vi "ATF-Sample Rate.vi"(10 "Sample Rate":T2, 11 "Device List":T3) -> ()   [LabVIEW 2022 SP3]
panel:
  out "SR":T1
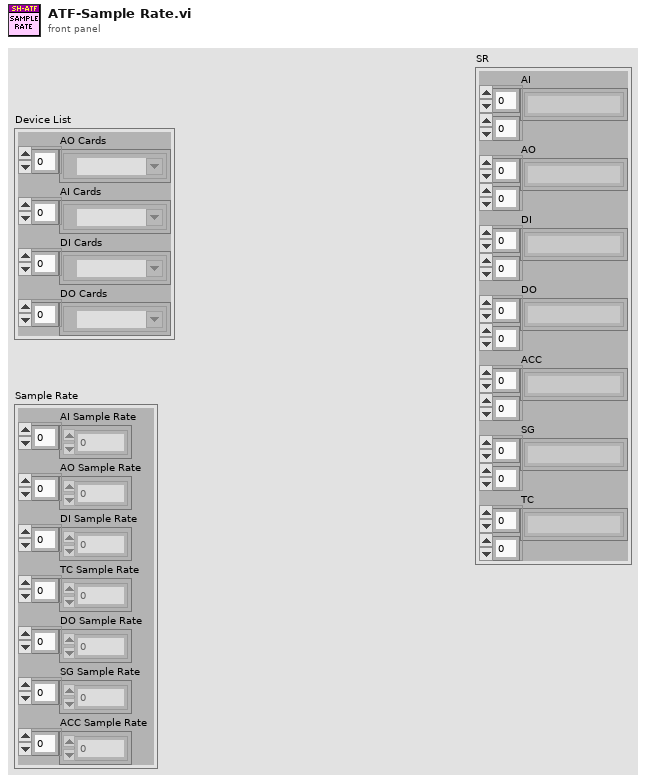
[diagram p1: front panel]
types:
  T1 = cluster{"AI":string[][], "AO":string[][], "DI":string[][], "DO":string[][], "ACC":string[][], "SG":string[][], "TC":string[][]}
  T2 = cluster{"AI Sample Rate":dbl[], "AO Sample Rate":dbl[], "DI Sample Rate":dbl[], "TC Sample Rate":dbl[], "DO Sample Rate":dbl[], "SG Sample Rate":dbl[], "ACC Sample Rate":dbl[]}
  T3 = cluster{"AO Cards":tag[], "AI Cards":tag[], "DI Cards":tag[], "DO Cards":tag[]}
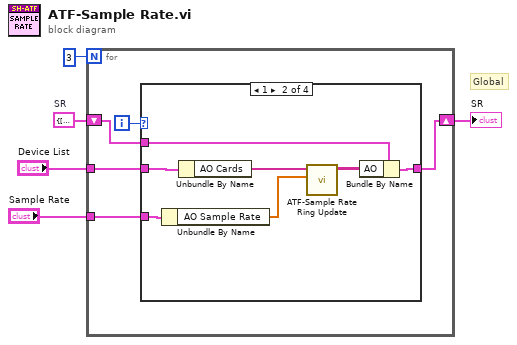
[diagram p0: block diagram]
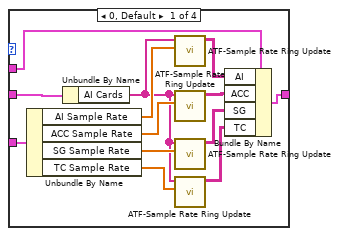
[diagram p2: hidden frame]
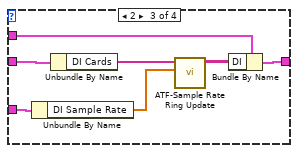
[diagram p3: hidden frame]
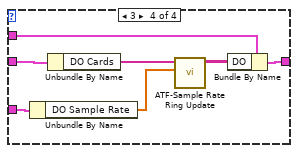
[diagram p4: hidden frame]
diagram:
  w2 = T1 {"AI"=[], "AO"=[], "DI"=[], "DO"=[], "ACC"=[], "SG"=[], "TC"=[]}  # SR
  # "Global"
  n1 = for {
    N: 3 -> [_]
    tunnel: "Device List" -> [w10]
    shift-right: [w7] -> w1
    shift-left: w2 -> [w8]
    tunnel: "Sample Rate" -> [w6]
    i -> [w9]
    n2 = case shown="1" w9 {
      tunnel: w10 -> [w23 w30 w37 w44]
      tunnel: w8 -> [w22 w28 w35 w42]
      tunnel: [w21 w27 w34 w41] -> w7
      tunnel: w6 -> [w20 w25 w32 w39]
      frame 0, Default {
        n3 = Unbundle By Name(w20) -> ("AI Sample Rate"=w19:dbl[], "ACC Sample Rate"=w18:dbl[], "SG Sample Rate"=w17:dbl[], "TC Sample Rate"=w16:dbl[])
        n4 = Unbundle By Name(w23) -> ("AI Cards"=w15:tag[])
        n5 = call "ATF-Sample Rate Ring Update.vi"("SR"=w19, "DL"=w15) -> ("Array"=w14:string[][])  [unwired: 9 in]
        n6 = call "ATF-Sample Rate Ring Update.vi"("SR"=w18, "DL"=w15) -> ("Array"=w13:string[][])  [unwired: 9 in]
        n7 = call "ATF-Sample Rate Ring Update.vi"("SR"=w17, "DL"=w15) -> ("Array"=w12:string[][])  [unwired: 9 in]
        n8 = call "ATF-Sample Rate Ring Update.vi"("SR"=w16, "DL"=w15) -> ("Array"=w11:string[][])  [unwired: 9 in]
        n9 = Bundle By Name(cluster=w22, "AI"=w14, "ACC"=w13, "SG"=w12, "TC"=w11) -> (w21:T1)
      }
      frame 1 {
        n10 = Unbundle By Name(w25) -> ("AO Sample Rate"=w24:dbl[])
        n11 = Unbundle By Name(w30) -> ("AO Cards"=w29:tag[])
        n12 = call "ATF-Sample Rate Ring Update.vi"("SR"=w24, "DL"=w29) -> ("Array"=w26:string[][])  [unwired: 9 in]
        n13 = Bundle By Name(cluster=w28, "AO"=w26) -> (w27:T1)
      }
      frame 2 {
        n14 = Unbundle By Name(w32) -> ("DI Sample Rate"=w31:dbl[])
        n15 = Unbundle By Name(w37) -> ("DI Cards"=w36:tag[])
        n16 = call "ATF-Sample Rate Ring Update.vi"("SR"=w31, "DL"=w36) -> ("Array"=w33:string[][])  [unwired: 9 in]
        n17 = Bundle By Name(cluster=w35, "DI"=w33) -> (w34:T1)
      }
      frame 3 {
        n18 = Unbundle By Name(w39) -> ("DO Sample Rate"=w38:dbl[])
        n19 = Unbundle By Name(w44) -> ("DO Cards"=w43:tag[])
        n20 = call "ATF-Sample Rate Ring Update.vi"("SR"=w38, "DL"=w43) -> ("Array"=w40:string[][])  [unwired: 9 in]
        n21 = Bundle By Name(cluster=w42, "DO"=w40) -> (w41:T1)
      }
    }
  }
  "SR" <- w1
